vi "S2C_STEP_FormatSettings.vi"(8 "Error In":errorcluster, 9 "Settings":string[](array[string]), 10 "Row":i32, 11 "Data In":string[][](array[string])) -> (0 "Error Out":errorcluster, 3 "Data Out":string[][](array[string]))   [LabVIEW 2015]
doc: "Updates the parameter value and adds the JSON text to the table row."
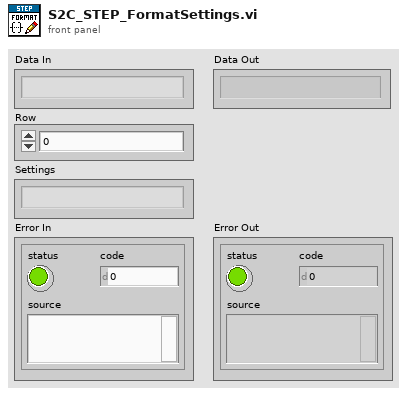
[diagram p1: front panel]
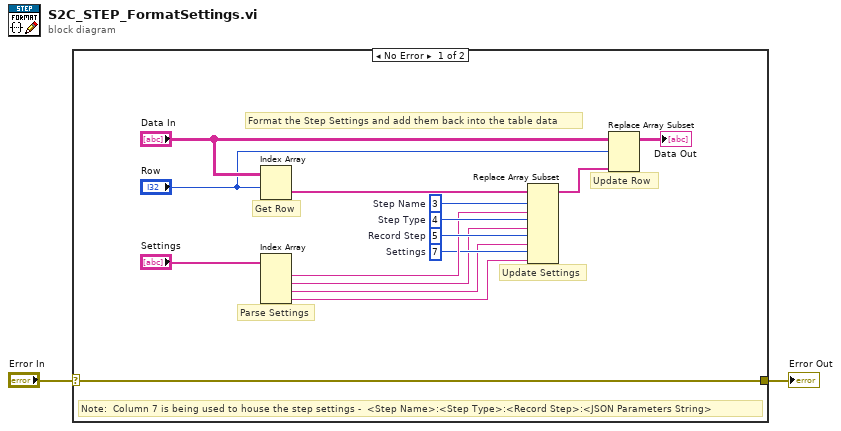
[diagram p0: block diagram]
diagram:
  n1 = case shown="No Error" "Error In" {
    selector: "Error In" -> [w17 w18]
    tunnel: [w17 w18] -> w1
    frame No Error {
      w7 = 7  # Settings
      w11 = 5  # Record Step
      w12 = 4  # Step Type
      w16 = 3  # Step Name
      # "Parse Settings"
      # "Note:  Column 7 is being used to house the step settings -  <Step Name>:<Step Type>:<Record Step>:<JSON Parameters String>"
      # "Update Row"
      # "Update Settings"
      # "Get Row"
      # "Format the Step Settings and add them back into the table data"
      n2 = Index Array(array="Data In", index (row)="Row") -> (element=w8:string[])  [unwired: 1 in]
      n3 = Index Array(array="Settings") -> (element #1=w10:string, element #2=w5:string, element #3=w3:string, element #4=w4:string)  [unwired: 4 in]
      n4 = Replace Array Subset(array=w8, new element #1=w10, index #1=w16, new element #2=w5, index #2=w12, new element #3=w3, index #3=w11, new element #4=w4, index #4=w7) -> (w9:string[])
      n5 = Replace Array Subset(array="Data In", new element=w9, index (row)="Row") -> (→"Data Out":string[][])  [unwired: 1 in]
    }
    frame Error {
    }
  }
  "Error Out" <- w1
